vi "Alpha Ver 1.4.vi"() -> ()   [LabVIEW 2015]
uses:
  <instrlib>/Keithley 622x LV 2009/Configure/Source/Typedefs/KE622x -- Current Range.ctl
  <instrlib>/Keithley 622x LV 2009/Configure/Source/Typedefs/KE622x -- Current Ranges.ctl
  <instrlib>/Keithley 622x LV 2009/Typedefs/KE622x -- On Off Control.ctl
  <instrlib>/Keithley 622x LV 2009/Utility/Typedefs/KE622x -- Instrument Type.ctl
  <instrlib>/Keithley 622x LV 2009/Configure/Source/Typedefs/KE622x -- Voltage Limit.ctl
  <instrlib>/Keithley 2000/Public/Configure/Configure DC Volts.vi
  <userlib>/LV-Link3/PolySubVIs/DtCreateAinChan.vi
  <userlib>/LV-Link3/PolySubVIs/DtOLReadMultipleSingle.vi
  <instrlib>/Keithley 2000/Keithley 2000.lvlib
  <instrlib>/Keithley 622x LV 2009/Keithley 622x.lvlib
panel:
  out "XTC":i32
  out "SEN":i32
  in  "Time Delay":u16(ring) items=["0.1", "1", "3", "10", "30", "60"]
  out "FILE":refnum<file>
  out "Tick":u32
  in  "MULTIPLE GRAPHS Y":u16(ring) items=["Linear", "Log"]
  in  "MULTIPLE GRAPHS X":u16(ring) items=["Linear", "Log"]
  in  "TIME GRAPH Y":u16(ring) items=["Linear", "Log"]
  in  "TIME GRAPH X":u16(ring) items=["Linear", "Log"]
  in  "Lock-In, Y":dbl=1.0
  in  "Lock-In, X":dbl=1.0
  in  "DAQ A4":dbl=1.0
  in  "DAQ A3":dbl=1.0
  in  "DAQ A2":dbl=1.0
  in  "DAQ A1":dbl=1.0
  in  "DAQ A0":dbl=1.0
  in  "2000":dbl=1.0
  in  "Current":dbl=1000.0
  in  "Display Type 3":u16(ring)=3 items=["X %", "Y %", "X Calibrated", "Y Calibrated", "Mag %", "Mag Calibrated", "Phase Degrees", "Ratio", "ADC 1", "ADC 2", "ADC 3", "ADC 4 ", "Noise %", "Noise Calibrated", "Ref Frequency", "", ""]
  in  "Display Type 2":u16(ring)=2 items=["X %", "Y %", "X Calibrated", "Y Calibrated", "Mag %", "Mag Calibrated", "Phase Degrees", "Ratio", "ADC 1", "ADC 2", "ADC 3", "ADC 4 ", "Noise %", "Noise Calibrated", "Ref Frequency", "", ""]
  out "Units 3":string
  out "Display 3":dbl format="%.3f"
  out "Units 2":string
  out "Display 2":dbl format="%.3f"
  out "DAQ A4":dbl format="%#_13g"
  out "DAQ_clust":T1
  out "DAQ A3":dbl format="%#_13g"
  out "DAQ A2":dbl format="%#_13g"
  out "DAQ A1":dbl format="%#_13g"
  out "Real stop cur":dbl format="%#_13g"
  out "Real start cur":dbl format="%#_13g"
  in  "Stop cur prefix":u16(ring)=2
  in  "Start cur prefix":u16(ring)=2
  out "MULTIPLE GRAPHS":cluster{dbl[], dbl[]}[](graph)
  in  "X-Axis":T2(ring)
  in  "Range":u8(ring)=20 items=["100nV", "200nV", "500nV", "1µV", "2µV", "5µV", "10µV", "20µV", "50µV", "100µV", "200µV", "500µV", "1mV", "2mV", "5mV", "10mV", "20mV", "50mV", "100mV", "200mV", "500mV", "1V"]
  in  "Display Type copy":u16(ring)=3 items=["X %", "Y %", "X Calibrated", "Y Calibrated", "Mag %", "Mag Calibrated", "Phase Degrees", "Ratio", "ADC 1", "ADC 2", "ADC 3", "ADC 4 ", "Noise %", "Noise Calibrated", "Ref Frequency", "", ""]
  out "Units copy":string
  out "Display copy":dbl format="%.3f"
  out "Overload":bool
  out "Display":dbl format="%.3f"
  out "Units":string
  in  "Display Type":u16(ring)=2 items=["X %", "Y %", "X Calibrated", "Y Calibrated", "Mag %", "Mag Calibrated", "Phase Degrees", "Ratio", "ADC 1", "ADC 2", "ADC 3", "ADC 4 ", "Noise %", "Noise Calibrated", "Ref Frequency", "", ""]
  in  "Time Constant":u16(ring) items=["MIN", "1ms", "3ms", "10ms", "30ms", "100ms", "300ms", "1s", "3s", "10s", "30s", "100s", "300s"]
  in  "Slope":u8(ring) items=["6db/octave", "12dB/octave"]
  in  "Dynamic Reserve":u16(ring) items=["High Stability", "Normal", "High Reserve"]
  in  "Auto Sensitivity":bool
  in  "Auto Measure":bool
  out "6221_error_out":errorcluster
  out "2000_error_out":errorcluster
  out "5110_error_out":errorcluster
  out "Input Mode":i32(ring) items=[" Voltage Input (A or A-B) ", "Current Input 10E6 V/A", "Current Input 10E8 V/A"]
  out "5110":refnum<visa-resource-name>
  in  "GPIB Address":i8=11 min=1 max=32 step=1
  out "DAQ A0":dbl format="%#_13g"
  out "2000":dbl format="%#_13g"
  in  "Device":string(combo)
  in  "Number \nof points":i32=10
  in  "Folder\nprename":string
  out "TIME GRAPH":cluster{dbl[], dbl[]}[](graph)
  out "T0":u32
  out "LIMIT":bool
  out "LIMIT":bool
  out "Error Code":string
  in  "Comments":string
  out "2000":refnum<visa-resource-name>
  out "6221":refnum<visa-resource-name>
  out "Step  (A)":dbl=5e-05 format="%#_3p"
  in  "Stop\ncurrent (A)":dbl=2.0 format="%#_6p"
  in  "Start \ncurrent (A)":dbl=1.0 format="%#_6p"
  in  "Check For SCPI Errors? (T)":bool=TRUE
  out "Interlock Tripped?":bool
  out "Compliance?":bool
  in  "Turn Off Output \nIf Compliance?":bool=TRUE
  in  "Turning ON/OFF\ncurrent output":T3=enum."On"
  in  "Range Selection":T4={"Auto Range?"=TRUE, "Man / Selected\nRange"=enum."2nA"}
  # "FILE CONFIGURATION"
  # "ADMIN PANEL"
  # "MULTIPLIERS"
  # "SCALES"
  # "KEITHLEY 6221 CONFIGURATION (ADMIN ONLY)"
  # "KEITHLEY DAQ CONFIGURATION (ADMIN ONLY)"
  # "PRINCETON LOCK-IN AMP (ADMIN ONLY)"
  # "I don't know what the hell it is,\njust don't touch it"
  # "SENSITIVITY"
  # "INPUT CONFIGURATION"
  # "READINGS"
  # "START, STOP, STEP, CONFIGURATION"
  # "IF ON"
  # "Output Channels Time - Constant \nSlope & Dynamic Reserve"
  # "Compliance = Limiting output voltage\nThis switch determines if we want to switch \noff the current output if wee exceed compliance"
  # "SCALES"
  # "LOCK-IN READINGS"
  # "RIGHT DISPLAY"
  # "LEFT DISPLAY"
  # "There is a safe switch at \nthe back of the instrument \nThis indicator shows if it is on"
  # "You have hit a damn jackpot \nby exceeding the limited voltage\nCongrats"
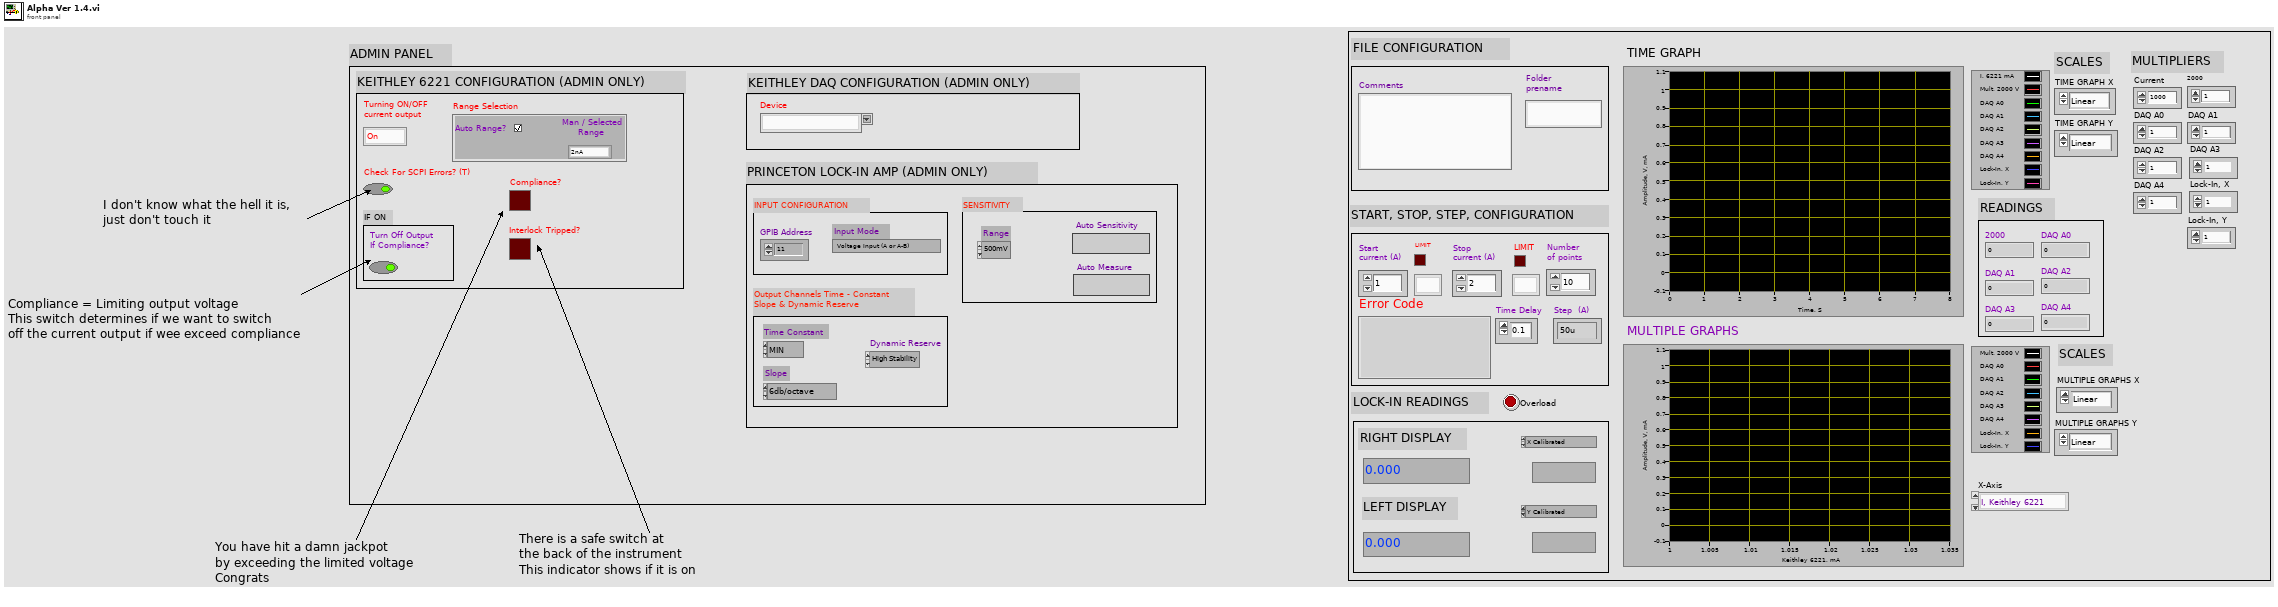
[diagram p1: front panel]
types:
  T1 = cluster{"Task out":i32, "Actual Number of Channels":u32, "error out":errorcluster}
  T2 = enum16{"I, Keithley 6221", "V, Keithley 2000", "V, Keithley DAQ A0", "V, Keithley DAQ A1", "V, Keithley DAQ A2", "V, Keithley DAQ A3", "V, Keithley DAQ A4", "V, Lock-In X", "V, Lock-In Y"}
  T3 = typedef "Keithley 622x.lvlib/KE622x -- On Off Control.ctl" = enum16{"Off", "On"}
  T4 = typedef "Keithley 622x.lvlib/KE622x -- Current Range.ctl" = cluster{"Auto Range?":bool, "Man / Selected\nRange":T5}
  T5 = typedef "Keithley 622x.lvlib/KE622x -- Current Ranges.ctl" = enum16{"2nA", "20nA", "200nA", "2uA", "20uA", "200uA", "2mA", "20mA", "100mA"}
  T6 = typedef "Keithley 622x.lvlib/KE622x -- Instrument Type.ctl" = enum16{"KE6220", "KE6221"}
  T7 = typedef "Keithley 622x.lvlib/KE622x -- Voltage Limit.ctl" = dbl
  T8 = cluster{"Task out":i32, "error out":errorcluster}
  T9 = cluster{dbl, dbl, dbl, dbl, dbl, "Measurement":dbl}
  T10 = cluster{dbl[], dbl[], dbl[], dbl[], dbl[], dbl[], dbl[], dbl[], dbl[], dbl[]}
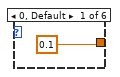
[diagram p2: hidden frame]
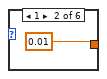
[diagram p3: hidden frame]
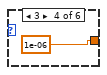
[diagram p4: hidden frame]
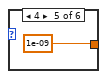
[diagram p5: hidden frame]
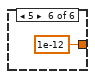
[diagram p6: hidden frame]
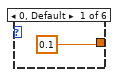
[diagram p7: hidden frame]
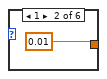
[diagram p8: hidden frame]
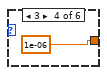
[diagram p9: hidden frame]
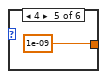
[diagram p10: hidden frame]
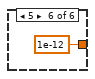
[diagram p11: hidden frame]
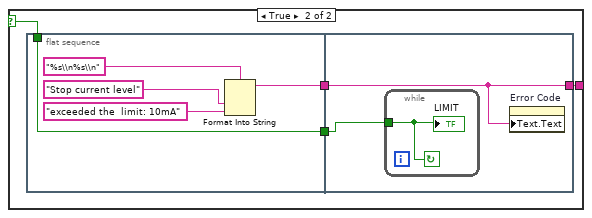
[diagram p12: hidden frame]
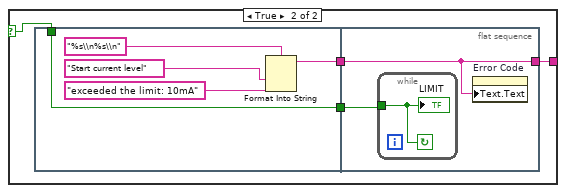
[diagram p13: hidden frame]
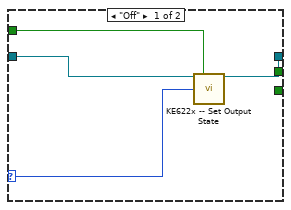
[diagram p14: hidden frame]
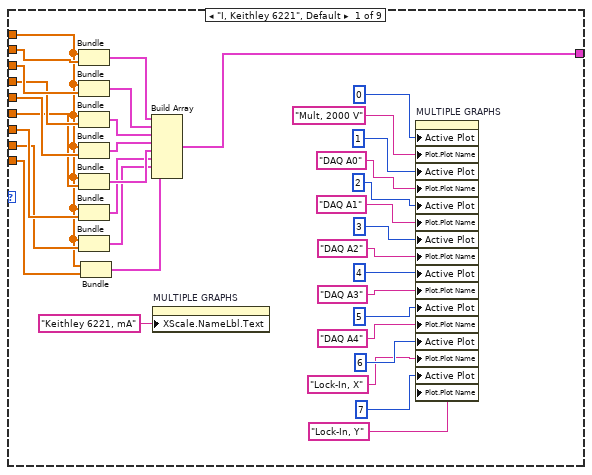
[diagram p15: hidden frame]
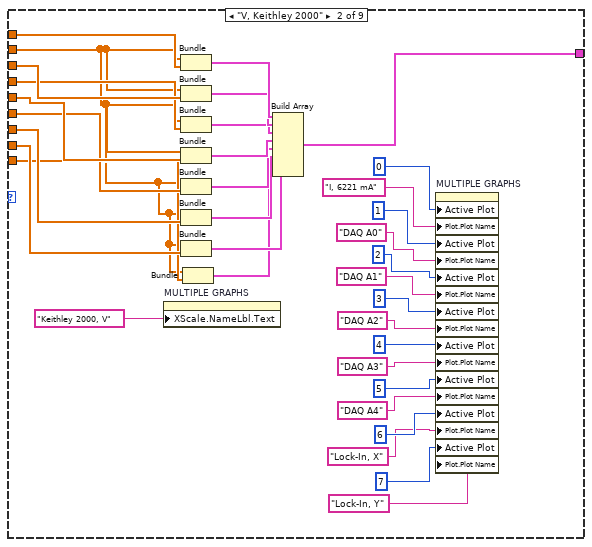
[diagram p16: hidden frame]
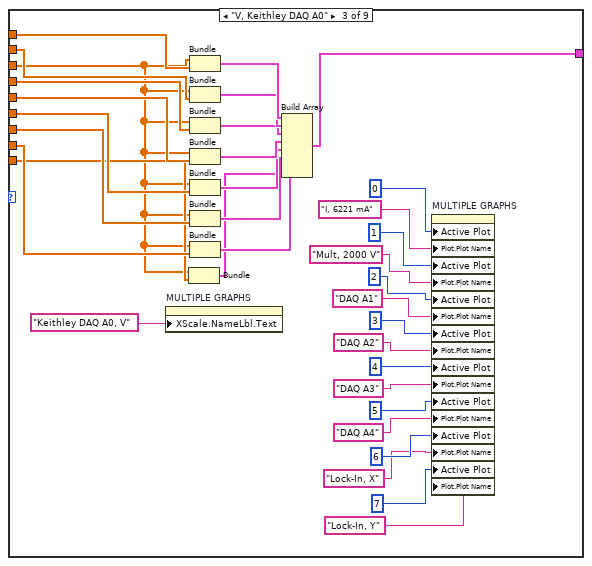
[diagram p17: hidden frame]
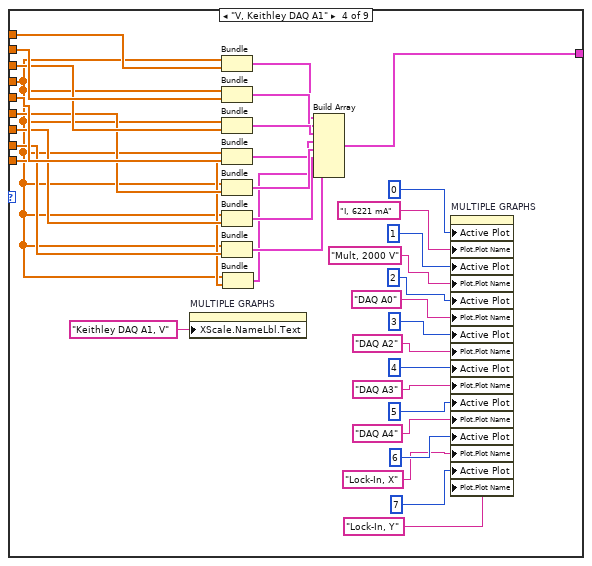
[diagram p18: hidden frame]
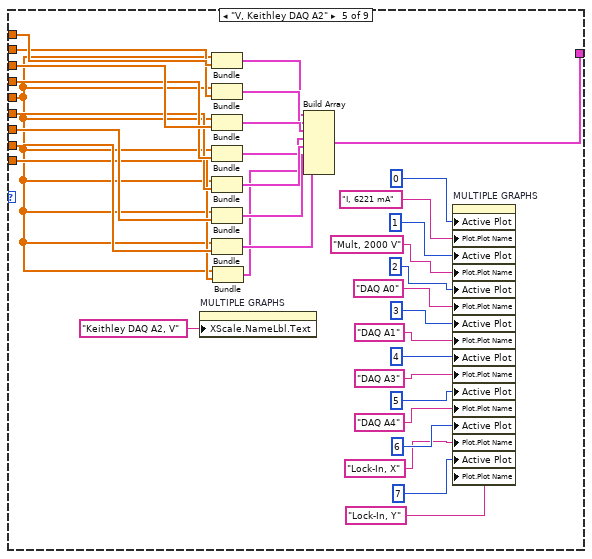
[diagram p19: hidden frame]
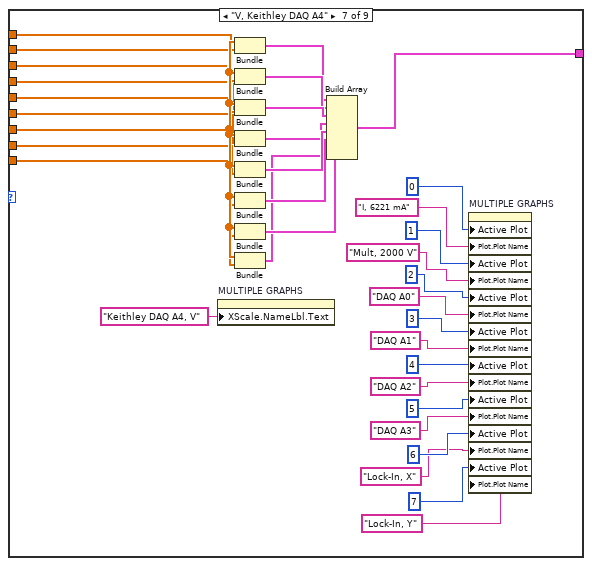
[diagram p20: hidden frame]
diagram:
  n1 = flat-sequence {
    tunnel: [w177] -> w7
    tunnel: [w176] -> w6
    tunnel: [w175] -> w5
    tunnel: [w174] -> w4
    tunnel: [w173] -> w3
    tunnel: [w172] -> w2
    tunnel: [w161] -> w1
    tunnel: w7 -> [w1027]
    tunnel: w6 -> [w1026]
    tunnel: w5 -> [w1025]
    tunnel: w4 -> [w1024]
    tunnel: w3 -> [w1023]
    tunnel: w2 -> [w1022]
    tunnel: w1 -> [w1021]
    frame #0 {
      # "File configuration"
      # "Start, Stop, Step"
      # "Initializing instruments"
      n2 = flat-sequence {
        frame #0 {
          w15 = TRUE  # reset
          w14 = FALSE  # ID query
          # "Initialize Lock-In 5110"
          # "Initialize Keithley 2000"
          # "Initialize Keithley 6221"
          n3 = call <instrlib>:"Initialize.vi"("VISA resource name"=refnum<visa-resource-name> "KEITHLEY_MULTIMETER") -> ("VISA resource name out"=w19:refnum<visa-resource-name>)  [unwired: 17 in, 1 out]
          n4 = call <instrlib>:"Initialize.vi"("VISA resource name"=refnum<visa-resource-name> "KEITHLEY_DC_AC_CURRENT_SOURCE", "Error Queue Option"=enum16{"Clear Error Queue", "Error Query"}."Clear Error Queue", "Instrument Type"=KE622x_--_Instrument_Type."KE6221") -> ("VISA resource name out"=→"6221":refnum<visa-resource-name>, "error out"=→"6221_error_out":errorcluster)  [unwired: 11 in]
          n5 = call "SR51XX Initialize"("VISA session (for class)"=refnum<visa-resource-name> "LOCK_IN_5110_PRINCETON", "Interface"=FALSE, "ID query"=w14, "GPIB Address"="GPIB Address", "reset"=w15) -> ("VISA session"=→"5110":refnum<visa-resource-name>, "error out"=→"5110_error_out":errorcluster)  [unwired: 8 in, 1 out]
          n6 = call-poly <instrlib>:"Configure Measurement.vi"("VISA resource name"=w19) -> ("VISA resource name out"=→"2000":refnum<visa-resource-name>, "error out"=→"2000_error_out":errorcluster)  [unwired: 17 in]
        }
        frame #1 {
          # "Initialize Keithley DAQ \n(getting board name)"
          n7 = call <userlib>:"DtOLGetBoardNames.vi"() -> ("Number of boards"=w24:u32)  [unwired: 9 in, 2 out]
          n8 = Initialize Array("", w24) -> (w26:string[])
          n9 = for {
            N: w24 -> [_]
            shift-right: [w32] -> w29
            shift-left: w26 -> [w33]
            i -> [w31]
            n10 = Add(x=1, y=w31) -> (x+y=w35:i32)
            n11 = call <userlib>:"DtOLGetBoardNames.vi"("Select Board"=w35) -> ("Board Name"=w30:string)  [unwired: 8 in, 2 out]
            n12 = Replace Array Subset(array=w33, new element=w30, index=w31) -> (w32:string[])
          }
          n13 = Index Array(array=w29, index=0) -> (element=w28:string)
          n14 = property on="Device" class="CmbBox"("Strings[]"=w29, "Value"=w28) -> ()  [unwired: 2 in, 2 out]
        }
        frame #2 {
          # "Calculating steps by number\nof points"
          # "Putting in a loop \ninstead of \"STOP\""
          n15 = local read "Real stop cur"() -> (w52:dbl)
          n16 = local read "Real start cur"() -> (w53:dbl)
          n17 = case shown="2" "Start cur prefix" {
            tunnel: [0.1 0.01 0.001 1e-06 1e-09 1e-12] -> w41
            frame 0, Default {
            }
            frame 1 {
            }
            frame 2 {
            }
            frame 3 {
            }
            frame 4 {
            }
            frame 5 {
            }
          }
          n18 = case shown="2" "Stop cur prefix" {
            tunnel: [0.1 0.01 0.001 1e-06 1e-09 1e-12] -> w39
            frame 0, Default {
            }
            frame 1 {
            }
            frame 2 {
            }
            frame 3 {
            }
            frame 4 {
            }
            frame 5 {
            }
          }
          n19 = Subtract(x=w52, y=w53) -> (x-y=w55:dbl)
          n20 = Multiply(x=w41, y="Start \ncurrent (A)") -> (x*y=w37:dbl)
          "Real start cur" <- w37
          n21 = Divide(x=w55, y="Number \nof points") -> (x/y=→"Step  (A)":dbl)
          n22 = Multiply(x=w39, y="Stop\ncurrent (A)") -> (x*y=w36:dbl)
          "Real stop cur" <- w36
          n23 = Greater?(x=w36, y=T7 0.01) -> (0:w47:bool)
          n24 = Greater?(x=w37, y=T7 0.01) -> (0:w46:bool)
          n25 = case shown="False" w47 {
            selector: w47 -> [_ w71]
            tunnel: [w68 w74] -> w49
            frame False {
              n26 = Format Into String(format string="%s\\n", "Start current level is OK" ("false string")) -> (resulting string=w68:string)  [unwired: 2 in, 1 out]
            }
            frame True {
              n27 = flat-sequence {
                tunnel: [w76] -> w73
                tunnel: [w75] -> w72
                tunnel: w71 -> [w75]
                tunnel: [w80] -> w74
                tunnel: w73 -> [w80]
                tunnel: w72 -> [w81]
                frame #0 {
                  n28 = Format Into String(format string="%s\\n%s\\n", "Stop current level" ("String"), "exceeded the  limit: 10mA" ("input 2")) -> (resulting string=w76:string)  [unwired: 2 in, 1 out]
                }
                frame #1 {
                  n29 = while {
                    tunnel: w81 -> [w82]
                    stop <- w82 continue-if-true
                    "LIMIT" <- w82
                  }
                  n30 = property on="Error Code" class="Str"("Text.Text"=w80) -> ()  [unwired: 2 in, 2 out]
                }
              }
            }
          }
          n31 = case shown="False" w46 {
            selector: w46 -> [_ w87]
            tunnel: [w83 w89] -> w48
            frame False {
              n32 = Format Into String(format string="%s\\n", "Start current level is OK" ("false string")) -> (resulting string=w83:string)  [unwired: 2 in, 1 out]
            }
            frame True {
              n33 = flat-sequence {
                tunnel: [w91] -> w88
                tunnel: w87 -> [w90]
                tunnel: [w90] -> w86
                tunnel: [w95] -> w89
                tunnel: w88 -> [w95]
                tunnel: w86 -> [w96]
                frame #0 {
                  n34 = Format Into String(format string="%s\\n%s\\n", "Start current level" ("String"), "exceeded the limit: 10mA" ("input 2")) -> (resulting string=w91:string)  [unwired: 2 in, 1 out]
                }
                frame #1 {
                  n35 = while {
                    tunnel: w96 -> [w97]
                    stop <- w97 continue-if-true
                    "LIMIT" <- w97
                  }
                  n36 = property on="Error Code" class="Str"("Text.Text"=w95) -> ()  [unwired: 2 in, 2 out]
                }
              }
            }
          }
          n37 = Concatenate Strings(w48, w49) -> (→"Error Code":string)
        }
        frame #3 {
          # "Adding headlines"
          # "Creating folder&file"
          # "Creating comments"
          # "Writing instr params"
          n38 = local read "5110"() -> (w103:refnum<visa-resource-name>)
          n39 = local read "Real stop cur"() -> (w101:dbl)
          n40 = local read "Real start cur"() -> (w102:dbl)
          n41 = call "folder_creation.vi"("Name"="Folder\nprename") -> ("String"=w119:string)
          n42 = call "file_creation.vi"("String"=w119) -> ("refnum out"=w104:refnum<file>)
          "FILE" <- w104
          n43 = call "com_inst.vi"("Stop current"=w101, "Start current"=w102, "VISA session (for class)"=w103) -> ("XTC"=→"XTC":i32, "SEN"=→"SEN":i32, "concatenated string"=w100:string)
          n44 = Format Into String(format string="# %s\\n", initial string=w104, "Comments") -> (resulting string=w106:refnum<file>)  [unwired: 1 in, 1 out]
          n45 = Format Into String(format string="# %s\\n", initial string=w106, w100) -> (resulting string=w105:refnum<file>)  [unwired: 1 in, 1 out]
          n46 = Format Into String(format string="# %-6s  %-12s %-12s %-14s %-12s %-14s %-12s %-12s %-14s%-14s\\n", initial string=w105, "t, ms" ("input 3"), "2000, V" ("input 1"), "DAQ A0, V" ("input 2"), "DAQ A1, V" ("input 2"), "DAQ A2, V" ("input 2"), "DAQ A3, V" ("input 2"), "DAQ A4, V" ("input 2"), "5110_X, V" ("input 3"), "5110_Y, V " ("input 3"), "6221, A" ("input 3")) -> ()  [unwired: 1 in, 2 out]
        }
        frame #4 {
          # "Time Intit"
          n47 = Wait Until Next ms Multiple(millisecond multiple=u32 1000) -> (millisecond timer value=→"T0":u32)
        }
      }
    }
    frame #1 {
      # "Configuring Keithley DAQ just before measuments"
      # "Configuring Keithley 6221 just before measuments"
      n48 = flat-sequence {
        tunnel: [w135] -> w125
        tunnel: [w153] -> _
        tunnel: [w155] -> _
        tunnel: w125 -> [w154]
        frame #0 {
          # "Current range \nselection check"
          # "Checking for compliance\nand interlock errors"
          n49 = local read "6221"() -> (w138:refnum<visa-resource-name>)
          n50 = call <instrlib>:"KE622x -- Set Current Range.vi"("Resource In"=w138, "Current Range In"="Range Selection", "Read Back Set Values? (T)"=FALSE) -> ("Resource Out (dupl)"=w143:refnum<visa-resource-name>)  [unwired: 10 in, 2 out]
          n51 = case shown="\"On\"" "Turning ON/OFF\ncurrent output" {
            selector: "Turning ON/OFF\ncurrent output" -> [w147 _]
            tunnel: [_ w151] -> w141
            tunnel: [_ w150] -> w142
            tunnel: "Check For SCPI Errors? (T)" -> [w146 _]
            tunnel: w143 -> [w144 w149]
            tunnel: [w145 w148] -> w135
            frame "Off" {
              n52 = call <instrlib>:"KE622x -- Set Output State.vi"("Resource In"=w144, "Check For SCPI Errors? (T)"=w146, "Output State"=w147) -> ("Resource Out (dupl)"=w145:refnum<visa-resource-name>)  [unwired: 11 in, 1 out]
            }
            frame "On" {
              n53 = call <instrlib>:"KE622x -- Turn Output On And Check For Errors.vi"("Resource In"=w149, "Turn Off Output If Compliance?"="Turn Off Output \nIf Compliance?") -> ("Resource Out (dupl)"=w148:refnum<visa-resource-name>, "Interlock Tripped?"=w151:bool, "Compliance?"=w150:bool)  [unwired: 10 in, 1 out]
            }
          }
          "Interlock Tripped?" <- w141
          "Compliance?" <- w142
        }
        frame #1 {
          # "Setting start current"
          n54 = local read "Real start cur"() -> (w153:dbl)
          n55 = Wait (ms)(milliseconds to wait=u32 100) -> ()  [unwired: 1 out]
          n56 = call <instrlib>:"KE622x -- Set Current Level.vi"("Resource In"=w154, "Current Level (A) In"=w153) -> ("Resource Out (dupl)"=w155:refnum<visa-resource-name>)  [unwired: 12 in, 1 out]
        }
      }
      n57 = flat-sequence {
        frame #0 {
          w130 = 100 items=["SingleEnded"=100, "Differential"=101] ("Channel Type")
          # "Configure the input channel"
          n58 = call-poly <userlib>:"DtOLCreateTask.vi"("Channel Type"=w130, "Range Min"=-10.0, "Range Max"=10.0, "Board Name"="Device", "Channel"="0:4" ("Channels")) -> ("Task out"=w129:i32, "Actual Number of Channels"=w128:u32, "error out"=w127:errorcluster)  [unwired: 8 in]
          n59 = Bundle("Task out"=w129, "Actual Number of Channels"=w128, "error out"=w127) -> (→"DAQ_clust":T1)  [unwired: 1 in]
        }
      }
    }
    frame #2 {
      n60 = local read "5110"() -> (w168:refnum<visa-resource-name>)
      n61 = local read "2000"() -> (w167:refnum<visa-resource-name>)
      n62 = local read "6221"() -> (w166:refnum<visa-resource-name>)
      n63 = local read "5110_error_out"() -> (w165:errorcluster)
      n64 = local read "6221_error_out"() -> (w164:errorcluster)
      n65 = local read "2000_error_out"() -> (w163:errorcluster)
      n66 = local read "DAQ_clust"() -> (w162:T1)
      n67 = while {
        shift-right: [w330] -> _
        shift-left: dbl[] [] -> [w455]
        shift-right: [w331] -> _
        shift-left: i32[] [] -> [w454]
        tunnel: w167 -> [w452]
        tunnel: w166 -> [w451]
        shift-right: [w288] -> _
        shift-left: dbl[] [] -> [w445]
        tunnel: [w444] -> w177
        tunnel: [w443] -> w176
        tunnel: [w441] -> w175
        tunnel: [w439] -> w174
        tunnel: w168 -> [w437]
        tunnel: w165 -> [w436]
        tunnel: w164 -> [w428]
        tunnel: w163 -> [w427]
        tunnel: [w392] -> w173
        tunnel: [w390] -> w172
        shift-right: [w290] -> _
        shift-left: dbl[] [] -> [w389]
        shift-right: [w291] -> _
        shift-left: dbl[] [] -> [w388]
        shift-right: [w332] -> _
        shift-left: dbl[] [] -> [w385]
        tunnel: w162 -> [w345]
        tunnel: [w344] -> w161
        shift-right: [w329] -> _
        shift-left: dbl[] [] -> [w343]
        shift-right: [w328] -> _
        shift-left: dbl[] [] -> [w342]
        shift-right: [w327] -> _
        shift-left: dbl[] [] -> [w341]
        shift-right: [w289] -> _
        shift-left: dbl[] [] -> [w293]
        i -> [w429]
        stop <- w446 stop-if-true
        # "V, DAQ A4"
        # "V, DAQ A3"
        # "V, DAQ A2"
        # "V, DAQ A1"
        # "Y-V, 5110"
        # "X-V, 5110"
        # "I, 6221"
        # "Config delay"
        # "Control subVI 5110"
        # "Read config 5110"
        # "Measurement config 5110"
        # "Time config 5110"
        # "Configuring Right Display 5110"
        # "Configuring Left Display 5110"
        # "Setting 6221 current"
        # "Delay before measuremens"
        # "Getting the data from DAQ and 2000"
        # "Changing input current"
        # "Time"
        # "V, DAQ A0"
        # "V, 2000"
        n68 = local read "T0"() -> (w453:u32)
        n69 = Quotient & Remainder(x=w429, y=10) -> (floor(x/y)=w434:i32)  [unwired: 1 out]
        n70 = Equal?(x=0, y=w429) -> (x = y?=w431:bool)
        n71 = Subtract(x=w420, y=w453) -> (x-y=w354:u32)
        n72 = Equal?(x=1, y=w434) -> (x = y?=w430:bool)
        n73 = Divide(x=w354, y=u32 1000) -> (x/y=w355:dbl)
        n74 = local read "FILE"() -> (w193:refnum<file>)
        n75 = flat-sequence {
          tunnel: w452 -> [w780]
          tunnel: [w780] -> w384
          tunnel: w451 -> [w779]
          tunnel: [w779] -> w382
          tunnel: w437 -> [w778]
          tunnel: [w778] -> w380
          tunnel: [w777] -> w378
          tunnel: w436 -> [w777]
          tunnel: w431 -> [w776]
          tunnel: [w776] -> w376
          tunnel: w430 -> [w775]
          tunnel: [w775] -> w374
          tunnel: w428 -> [w774]
          tunnel: [w774] -> w372
          tunnel: w427 -> [w773]
          tunnel: [w773] -> w370
          tunnel: [w771] -> w420
          tunnel: [w772] -> w346
          tunnel: w345 -> [w772]
          tunnel: w384 -> [w795]
          tunnel: [w795] -> w383
          tunnel: w382 -> [w794]
          tunnel: [w794] -> w381
          tunnel: w380 -> [w793]
          tunnel: [w793] -> w379
          tunnel: w378 -> [w792]
          tunnel: [w792] -> w377
          tunnel: w376 -> [w791]
          tunnel: [w791] -> w375
          tunnel: w374 -> [w790]
          tunnel: [w790] -> w373
          tunnel: w372 -> [w789]
          tunnel: [w789] -> w371
          tunnel: w370 -> [w788]
          tunnel: [w788] -> w369
          tunnel: [w781] -> w347
          tunnel: w346 -> [w781]
          tunnel: w383 -> [w808]
          tunnel: [w808] -> w419
          tunnel: w381 -> [w807]
          tunnel: [w807] -> w418
          tunnel: w379 -> [w806]
          tunnel: w377 -> [w803]
          tunnel: [w802] -> w417
          tunnel: [w801] -> w416
          tunnel: w375 -> [w800]
          tunnel: [w800] -> w415
          tunnel: w373 -> [w799]
          tunnel: w371 -> [w798]
          tunnel: [w798] -> w414
          tunnel: w369 -> [w797]
          tunnel: [w797] -> w413
          tunnel: [w796] -> w348
          tunnel: w347 -> [w796]
          tunnel: w419 -> [w833]
          tunnel: [w833] -> w412
          tunnel: w418 -> [w832]
          tunnel: [w832] -> w411
          tunnel: w417 -> [w829]
          tunnel: [w828] -> w410
          tunnel: w416 -> [w827]
          tunnel: [w826] -> w409
          tunnel: w415 -> [w824]
          tunnel: [w824] -> w408
          tunnel: w414 -> [w831]
          tunnel: [w831] -> w407
          tunnel: w413 -> [w830]
          tunnel: [w830] -> w406
          tunnel: ["Auto Measure"] -> w405
          tunnel: ["Auto Sensitivity"] -> w404
          tunnel: [w819] -> w403
          tunnel: [w816] -> w349
          tunnel: w348 -> [w816]
          tunnel: w412 -> [w852]
          tunnel: [w852] -> w368
          tunnel: w411 -> [w851]
          tunnel: [w851] -> w367
          tunnel: w410 -> [w844]
          tunnel: w409 -> [w842]
          tunnel: [w841] -> w366
          tunnel: w408 -> [w848]
          tunnel: [w848] -> w365
          tunnel: w407 -> [w850]
          tunnel: [w850] -> w364
          tunnel: w406 -> [w849]
          tunnel: [w849] -> w363
          tunnel: w405 -> [w846]
          tunnel: [w846] -> w362
          tunnel: w404 -> [w847]
          tunnel: [w847] -> w361
          tunnel: w403 -> [w837]
          tunnel: [w837] -> w360
          tunnel: [w843] -> w359
          tunnel: ["Time Constant"] -> w358
          tunnel: ["Slope"] -> w357
          tunnel: [w834] -> w350
          tunnel: w349 -> [w834]
          tunnel: [w874] -> w286
          tunnel: [w873] -> w285
          tunnel: [w859] -> w284
          tunnel: [w872] -> w283
          tunnel: [w871] -> w282
          tunnel: [w870] -> w281
          tunnel: [w869] -> w280
          tunnel: [w868] -> w279
          tunnel: [w861] -> w278
          tunnel: [w864] -> w277
          tunnel: [w862] -> w276
          tunnel: [w867] -> w275
          tunnel: w357 -> [w867]
          tunnel: w358 -> [w862]
          tunnel: w359 -> [w865]
          tunnel: w360 -> [w861]
          tunnel: w361 -> [w868]
          tunnel: w362 -> [w869]
          tunnel: w363 -> [w870]
          tunnel: w364 -> [w871]
          tunnel: w365 -> [w872]
          tunnel: w366 -> [w860]
          tunnel: w367 -> [w873]
          tunnel: w368 -> [w874]
          tunnel: [w853] -> w274
          tunnel: w350 -> [w853]
          tunnel: w286 -> [w897]
          tunnel: [w897] -> w273
          tunnel: w285 -> [w896]
          tunnel: [w896] -> w271
          tunnel: w284 -> [w888]
          tunnel: [w887] -> w269
          tunnel: w283 -> [w895]
          tunnel: [w895] -> w267
          tunnel: w282 -> [w894]
          tunnel: [w894] -> w265
          tunnel: w281 -> [w893]
          tunnel: [w893] -> w263
          tunnel: w280 -> [w892]
          tunnel: [w892] -> w261
          tunnel: w279 -> [w891]
          tunnel: [w891] -> w259
          tunnel: w278 -> [w882]
          tunnel: [w882] -> w257
          tunnel: w277 -> [w889]
          tunnel: [w886] -> w255
          tunnel: w276 -> [w884]
          tunnel: [w884] -> w253
          tunnel: w275 -> [w881]
          tunnel: [w881] -> w251
          tunnel: w274 -> [w890]
          tunnel: [w890] -> w249
          tunnel: [w877] -> w246
          tunnel: w273 -> [w920]
          tunnel: [w920] -> w272
          tunnel: w271 -> [w919]
          tunnel: [w919] -> w270
          tunnel: w269 -> [w910]
          tunnel: [w909] -> w268
          tunnel: w267 -> [w918]
          tunnel: [w918] -> w266
          tunnel: w265 -> [w917]
          tunnel: [w917] -> w264
          tunnel: w263 -> [w916]
          tunnel: [w916] -> w262
          tunnel: w261 -> [w915]
          tunnel: [w915] -> w260
          tunnel: w259 -> [w914]
          tunnel: [w914] -> w258
          tunnel: w257 -> [w905]
          tunnel: [w905] -> w256
          tunnel: w255 -> [w912]
          tunnel: [w911] -> w254
          tunnel: w253 -> [w907]
          tunnel: [w907] -> w252
          tunnel: w251 -> [w904]
          tunnel: [w904] -> w250
          tunnel: w249 -> [w913]
          tunnel: [w913] -> w248
          tunnel: [w900] -> w247
          tunnel: w272 -> [w942]
          tunnel: [w942] -> w402
          tunnel: w270 -> [w941]
          tunnel: [w941] -> w401
          tunnel: w268 -> [w928]
          tunnel: w266 -> [w940]
          tunnel: [w940] -> w400
          tunnel: w264 -> [w939]
          tunnel: [w939] -> w399
          tunnel: w262 -> [w938]
          tunnel: [w938] -> w398
          tunnel: w260 -> [w937]
          tunnel: [w937] -> w397
          tunnel: w258 -> [w936]
          tunnel: [w936] -> w396
          tunnel: w256 -> [w929]
          tunnel: w254 -> [w926]
          tunnel: [w925] -> w395
          tunnel: w252 -> [w930]
          tunnel: w250 -> [w931]
          tunnel: [w927] -> w394
          tunnel: [w924] -> w393
          tunnel: [w921] -> w351
          tunnel: w248 -> [w921]
          tunnel: [w946] -> w450
          tunnel: w429 -> [w954]
          tunnel: [w950] -> w446
          tunnel: [w944] -> w448
          tunnel: [w952] -> w447
          tunnel: [w949] -> w426
          tunnel: [w948] -> w425
          tunnel: [w947] -> w424
          tunnel: [w945] -> w423
          tunnel: [w944] -> w340
          tunnel: w393 -> [_]
          tunnel: w394 -> [w947]
          tunnel: w395 -> [w945]
          tunnel: w396 -> [_]
          tunnel: w397 -> [_]
          tunnel: w398 -> [w949]
          tunnel: w399 -> [w948]
          tunnel: w400 -> [_]
          tunnel: w401 -> [w952]
          tunnel: w402 -> [w946]
          tunnel: [w943] -> w352
          tunnel: w351 -> [w943]
          tunnel: w450 -> [w967]
          tunnel: [w967] -> w449
          tunnel: w448 -> [w966]
          tunnel: w447 -> [w965]
          tunnel: [w964] -> w442
          tunnel: [w963] -> w440
          tunnel: w426 -> [w961]
          tunnel: w425 -> [w962]
          tunnel: w424 -> [w959]
          tunnel: w423 -> [w960]
          tunnel: [w961] -> w422
          tunnel: [w960] -> w421
          tunnel: [w959] -> w391
          tunnel: [w958] -> w353
          tunnel: w352 -> [w958]
          tunnel: [w1004] -> w315
          tunnel: [w971] -> w314
          tunnel: [w1003] -> w313
          tunnel: [w1002] -> w312
          tunnel: [w1001] -> w311
          tunnel: [w1000] -> w310
          tunnel: [w972] -> w309
          tunnel: [w1004] -> w308
          tunnel: [w999] -> w307
          tunnel: [w998] -> w306
          tunnel: [w997] -> w305
          tunnel: [w970] -> w304
          tunnel: [w969] -> w303
          tunnel: [w968] -> w302
          tunnel: w353 -> [w994]
          tunnel: w391 -> [w998]
          tunnel: w421 -> [w999]
          tunnel: w422 -> [w995]
          tunnel: w440 -> [w1000]
          tunnel: w442 -> [w1001]
          tunnel: w449 -> [w996]
          tunnel: [w1008] -> w344
          tunnel: [w1009] -> w390
          tunnel: [w1010] -> w392
          tunnel: [w1011] -> w438
          tunnel: [w1012] -> w301
          tunnel: [w1013] -> w439
          tunnel: [w1014] -> w441
          tunnel: [w1015] -> w443
          tunnel: [w1016] -> w444
          tunnel: [w1017] -> w300
          tunnel: [w1018] -> w296
          tunnel: w315 -> [w1018]
          tunnel: w314 -> [w1017]
          tunnel: w313 -> [w1016]
          tunnel: w312 -> [w1015]
          tunnel: w311 -> [w1014]
          tunnel: w310 -> [w1013]
          tunnel: w309 -> [w1012]
          tunnel: w308 -> [w1011]
          tunnel: w307 -> [w1010]
          tunnel: w306 -> [w1009]
          tunnel: w305 -> [w1008]
          tunnel: [w1007] -> w299
          tunnel: w304 -> [w1007]
          tunnel: [w1006] -> w298
          tunnel: w303 -> [w1006]
          tunnel: w302 -> [w1005]
          tunnel: [w1005] -> w297
          frame #0 {
            n76 = Tick Count (ms)() -> (millisecond timer value=w771:u32)
            "Tick" <- w771
          }
          frame #1 {
            n77 = control-ref of="Range"() -> (w787:refnum<vi>)
            n78 = control-ref of="Auto Sensitivity"() -> (w786:refnum<vi>)
            n79 = control-ref of="Auto Measure"() -> (w785:refnum<vi>)
            n80 = control-ref of="Time Constant"() -> (w782:refnum<vi>)
            n81 = control-ref of="Slope"() -> (w783:refnum<vi>)
            n82 = control-ref of="Dynamic Reserve"() -> (w784:refnum<vi>)
            n83 = call "cont_ver_1.0.vi"("Dynamic Reserve"=w784, "Slope"=w783, "Time Constant"=w782, "Auto Measure"=w785, "Auto Sensitivity"=w786, "Range"=w787) -> ()
          }
          frame #2 {
            n84 = case shown="False" w799 {
              tunnel: w806 -> [w810 w815]
              tunnel: [w809 w813] -> w805
              tunnel: [w810 w812] -> w804
              tunnel: w803 -> [w809 w811]
              frame False {
              }
              frame True {
                n85 = call "SR51XX Read Preamp Input Mode"("VISA session (for class)"=w815, "error in (no error)"=w811) -> ("VISA session"=w812:refnum<visa-resource-name>, "Input Mode"=w814:i32, "error out"=w813:errorcluster)  [unwired: 15 in]
                n86 = local write "Input Mode"(w814) -> ()
              }
            }
            n87 = call "SR51XX Configure Signal Channel Input"("VISA session (for class)"=w804, "error in (no error)"=w805, "Update"=w800) -> ("VISA session"=w802:refnum<visa-resource-name>, "error out"=w801:errorcluster)  [unwired: 15 in]
          }
          frame #3 {
            n88 = local read "Input Mode"() -> (w825:i32)
            n89 = call "SR51XX Configure Sensitivity"("VISA session (for class)"=w829, "Input Mode"=w825, "Range"="Range", "error in (no error)"=w827, "Auto Sensitivity"="Auto Sensitivity", "Auto Measure"="Auto Measure", "Update"=w824) -> ("Range Annotations Out[]"=w817:string[], "VISA session"=w828:refnum<visa-resource-name>, "Auto Sensitivity out"=w821:bool, "Auto Measure out"=w820:bool, "Range Out"=w819:u8, "error out"=w826:errorcluster)  [unwired: 7 in]
            n90 = property on="Range" class="Ring (strict)"("Strings []"=w817) -> ()  [unwired: 2 in, 2 out]
            n91 = local write "Auto Sensitivity"(w821) -> ()
            n92 = local write "Auto Measure"(w820) -> ()
            n93 = local write "Range"(w819) -> ()
          }
          frame #4 {
            n94 = Or(x=w847, y=w846) -> (x .or. y?=w845:bool)
            n95 = call "SR51XX Configure Output Channels - Slope, TC and Dyn Reserve"("VISA session (for class)"=w844, "Time Constant"="Time Constant", "Slope"="Slope", "Check TC"=w845, "Dynamic Reserve"="Dynamic Reserve", "error in (no error)"=w842, "Range"=w837, "Update"=w848) -> ("VISA session"=w843:refnum<visa-resource-name>, "Slope Out"=w838:u8, "Time Constant Out"=w839:u16, "error out"=w841:errorcluster)  [unwired: 8 in]
            n96 = local write "Slope"(w838) -> ()
            n97 = local write "Time Constant"(w839) -> ()
          }
          frame #5 {
            n98 = local read "Input Mode"() -> (w866:i32)
            n99 = call "SR5110 Read Output"("VISA session (for class)"=w865, "Input Mode"=w866, "Time Constant"=w862, "Display Type"="Display Type", "Range"=w861, "error in (no error)"=w860, "Slope"=w867) -> ("Units"=→"Units":string, "Display Precision"=w858:i32, "Display"=→"Display":dbl, "VISA session"=w864:refnum<visa-resource-name>, "Available Display Types Out"=w857:string[], "Overload"=→"Overload":bool, "error out"=w859:errorcluster)  [unwired: 4 in, 2 out]
            n100 = property on="Display Type" class="Ring (strict)"("Strings []"=w857) -> ()  [unwired: 2 in, 2 out]
            n101 = property on="Display" class="DigNum (strict)"("Precision"=w858) -> ()  [unwired: 2 in, 2 out]
          }
          frame #6 {
            n102 = local read "Input Mode"() -> (w885:i32)
            n103 = call "SR5110 Read Output"("VISA session (for class)"=w889, "Input Mode"=w885, "Time Constant"=w884, "Display Type"="Display Type 2", "Range"=w882, "error in (no error)"=w888, "Slope"=w881) -> ("Units"=w875:string, "Display Precision"=w879:i32, "Display"=w876:dbl, "VISA session"=w886:refnum<visa-resource-name>, "Available Display Types Out"=w880:string[], "error out"=w887:errorcluster)  [unwired: 4 in, 3 out]
            "Display 2" <- w876
            "Units 2" <- w875
            n104 = call "pref_to_num.vi"("string"=w875) -> ("Numeric"=w878:dbl)
            n105 = property on="Display Type 2" class="Ring (strict)"("Strings []"=w880) -> ()  [unwired: 2 in, 2 out]
            n106 = property on="Display 2" class="DigNum (strict)"("Precision"=w879) -> ()  [unwired: 2 in, 2 out]
            n107 = Multiply(x=w878, y=w876) -> (x*y=w877:dbl)
          }
          frame #7 {
            n108 = local read "Input Mode"() -> (w908:i32)
            n109 = call "SR5110 Read Output"("VISA session (for class)"=w912, "Input Mode"=w908, "Time Constant"=w907, "Display Type"="Display Type 3", "Range"=w905, "error in (no error)"=w910, "Slope"=w904) -> ("Units"=w899:string, "Display Precision"=w903:i32, "Display"=w898:dbl, "VISA session"=w911:refnum<visa-resource-name>, "Available Display Types Out"=w902:string[], "error out"=w909:errorcluster)  [unwired: 4 in, 3 out]
            "Display 3" <- w898
            "Units 3" <- w899
            n110 = property on="Display 3" class="DigNum (strict)"("Precision"=w903) -> ()  [unwired: 2 in, 2 out]
            n111 = call "pref_to_num.vi"("string"=w899) -> ("Numeric"=w901:dbl)
            n112 = property on="Display Type 3" class="Ring (strict)"("Strings []"=w902) -> ()  [unwired: 2 in, 2 out]
            n113 = Multiply(x=w901, y=w898) -> (x*y=w900:dbl)
          }
          frame #8 {
            n114 = local read "Input Mode"() -> (w935:i32)
            n115 = call "SR5110 Read Output"("VISA session (for class)"=w926, "Input Mode"=w935, "Time Constant"=w930, "Display Type"="Display Type copy", "Range"=w929, "error in (no error)"=w928, "Slope"=w931) -> ("Units"=→"Units copy":string, "Display Precision"=w932:i32, "Display"=→"Display copy":dbl, "VISA session"=w925:refnum<visa-resource-name>, "Reference Unlock"=w924:bool, "Available Display Types Out"=w933:string[], "error out"=w927:errorcluster)  [unwired: 4 in, 2 out]
            n116 = property on="Display Type copy" class="Ring (strict)"("Strings []"=w933) -> ()  [unwired: 2 in, 2 out]
            n117 = property on="Display copy" class="DigNum (strict)"("Precision"=w932) -> ()  [unwired: 2 in, 2 out]
          }
          frame #9 {
            n118 = local read "Step  (A)"() -> (w955:dbl)
            n119 = local read "Real start cur"() -> (w956:dbl)
            n120 = Multiply(x=w955, y=w954) -> (x*y=w953:dbl)
            n121 = Add(x=w956, y=w953) -> (x+y=w944:dbl)
            n122 = local read "Real stop cur"() -> (w951:dbl)
            n123 = Greater Or Equal?(x=w944, y=w951) -> (x >= y?=w950:bool)
          }
          frame #10 {
            n124 = call <instrlib>:"KE622x -- Set Current Level.vi"("Resource In"=w965, "Current Level (A) In"=w966, "error in (no error)"=w962) -> ("Resource Out (dupl)"=w963:refnum<visa-resource-name>, "error out"=w964:errorcluster)  [unwired: 11 in]
            n125 = Wait Until Next ms Multiple(millisecond multiple=u32 50) -> ()  [unwired: 1 out]
          }
          frame #11 {
            n126 = Unbundle(w994) -> ("Task out"=w993:i32, "Actual Number of Channels"=w991:u32, "error out"=w992:errorcluster)
            n127 = call <instrlib>:"Data Read Single.vi"("VISA resource name"=w996, "error in (no error)"=w995) -> ("VISA resource name out"=w1002:refnum<visa-resource-name>, "Measurement"=w1004:dbl, "error out"=w1003:errorcluster)  [unwired: 13 in, 2 out]
            n128 = call-poly <userlib>:"DtOLRead.vi"("Number Chan to Read"=w991, "error in (no error)"=w992, "Task in"=w993) -> ("error out"=w989:errorcluster, "2D Data out"=w988:dbl[][], "Task out"=w990:i32)  [unwired: 4 in, 2 out]
            n129 = Index Array(array=w988, index (row) #1=0 ("index (row)"), index (row) #2=1 ("index (row)"), index (row) #3=2 ("index (row)"), index (row) #4=3 ("index (row)"), index (row) #5=4 ("index (row)")) -> (element #1=w987:dbl[], element #2=w981:dbl[], element #3=w980:dbl[], element #4=w979:dbl[], element #5=w978:dbl[])  [unwired: 5 in]
            n130 = Index Array(array=w978, index=0) -> (element=w968:dbl)
            n131 = Index Array(array=w987, index=0) -> (element=w972:dbl)
            n132 = Index Array(array=w981, index=0) -> (element=w971:dbl)
            n133 = Index Array(array=w980, index=0) -> (element=w970:dbl)
            n134 = Index Array(array=w979, index=0) -> (element=w969:dbl)
            n135 = Bundle("Task out"=w990, "error out"=w989) -> (w997:T8)  [unwired: 1 in]
          }
          frame #12 {
          }
        }
        n136 = Build Array (concatenate)(w454, w355) -> (w338:dbl[])
        n137 = property on="TIME GRAPH" class="XYGraph (strict)"("XScale.Mapping Mode"="TIME GRAPH X", "YScale.Mapping Mode"="TIME GRAPH Y") -> ()  [unwired: 2 in, 2 out]
        n138 = property on="MULTIPLE GRAPHS" class="XYGraph (strict)"("XScale.Mapping Mode"="MULTIPLE GRAPHS X", "YScale.Mapping Mode"="MULTIPLE GRAPHS Y") -> ()  [unwired: 2 in, 2 out]
        n139 = Bundle(w340, w246, w247) -> (w199:cluster{dbl, dbl, dbl})  [unwired: 1 in]
        n140 = Unbundle(w199) -> (w243:dbl, w209:dbl, w204:dbl)
        n141 = Unbundle(w199) -> (w184:dbl, w186:dbl, w185:dbl)
        n142 = Multiply(x=w243, y="Current") -> (x*y=w242:dbl)
        n143 = Multiply(x=w204, y="Lock-In, Y") -> (x*y=w205:dbl)
        n144 = Multiply(x=w209, y="Lock-In, X") -> (x*y=w210:dbl)
        n145 = Build Array (concatenate)(w385, w242) -> (w339:dbl[])
        n146 = Build Array (concatenate)(w389, w210) -> (w295:dbl[])
        n147 = Build Array (concatenate)(w388, w205) -> (w294:dbl[])
        n148 = Bundle(w301, w300, w299, w298, w297, "Measurement"=w296) -> (w316:T9)  [unwired: 1 in]
        n149 = Unbundle(w316) -> (w235:dbl, w229:dbl, w224:dbl, w219:dbl, w214:dbl, "Measurement"=w238:dbl)
        n150 = Unbundle(w316) -> (w191:dbl, w190:dbl, w189:dbl, w188:dbl, w187:dbl, "Measurement"=w192:dbl)
        n151 = Format Into String(format string="%08d  %8.2e %12g %14.5e %12.4e %12.4e  %12.4e %12.4e  %12.4e  %12g \\n", initial string=w193, w354, w192, w191, w190, w189, w188, w187, w186, w185, w184) -> ()  [unwired: 1 in, 2 out]
        n152 = Multiply(x=w238, y="2000") -> (x*y=w236:dbl)
        n153 = Multiply(x=w229, y="DAQ A1") -> (x*y=w230:dbl)
        n154 = Multiply(x=w235, y="DAQ A0") -> (x*y=w234:dbl)
        n155 = Multiply(x="DAQ A2", y=w224) -> (x*y=w225:dbl)
        n156 = Multiply(x=w214, y="DAQ A4") -> (x*y=w215:dbl)
        n157 = Multiply(x=w219, y="DAQ A3") -> (x*y=w220:dbl)
        n158 = Build Array (concatenate)(w455, w236) -> (w337:dbl[])
        n159 = Build Array (concatenate)(w343, w234) -> (w336:dbl[])
        n160 = Build Array (concatenate)(w342, w230) -> (w335:dbl[])
        n161 = Build Array (concatenate)(w341, w225) -> (w334:dbl[])
        n162 = Build Array (concatenate)(w445, w220) -> (w333:dbl[])
        n163 = Build Array (concatenate)(w293, w215) -> (w292:dbl[])
        n164 = Bundle(w339, w338, w337, w336, w335, w334, w333, w292, w295, w294) -> (w326:T10)  [unwired: 1 in]
        n165 = Unbundle(w326) -> (w244:dbl[], w202:dbl[], w241:dbl[], w232:dbl[], w227:dbl[], w222:dbl[], w217:dbl[], w211:dbl[], w207:dbl[], w201:dbl[])
        n166 = Bundle(w202, w244) -> (w245:cluster{dbl[], dbl[]})  [unwired: 1 in]
        n167 = Bundle(w202, w241) -> (w240:cluster{dbl[], dbl[]})  [unwired: 1 in]
        n168 = Bundle(w202, w232) -> (w231:cluster{dbl[], dbl[]})  [unwired: 1 in]
        n169 = Bundle(w202, w227) -> (w226:cluster{dbl[], dbl[]})  [unwired: 1 in]
        n170 = Bundle(w202, w217) -> (w216:cluster{dbl[], dbl[]})  [unwired: 1 in]
        n171 = Bundle(w202, w222) -> (w221:cluster{dbl[], dbl[]})  [unwired: 1 in]
        n172 = Bundle(w202, w211) -> (w212:cluster{dbl[], dbl[]})  [unwired: 1 in]
        n173 = Bundle(w202, w207) -> (w206:cluster{dbl[], dbl[]})  [unwired: 1 in]
        n174 = Bundle(w202, w201) -> (w200:cluster{dbl[], dbl[]})  [unwired: 1 in]
        n175 = Build Array(w245, w240, w231, w226, w221, w216, w212, w206, w200) -> (→"TIME GRAPH":cluster{dbl[], dbl[]}[])
        n176 = Unbundle(w326) -> (w325:dbl[], w324:dbl[], w323:dbl[], w322:dbl[], w321:dbl[], w320:dbl[], w319:dbl[], w318:dbl[], w287:dbl[])  [unwired: 1 out]
        n177 = case shown="\"V, Keithley DAQ A3\"" "X-Axis" {
          tunnel: [w475 w517 w552 w580 w622 w657 w692 w717 w752] -> w317
          tunnel: w325 -> [w472 w516 w551 w587 w621 w656 w690 w725 w760]
          tunnel: w324 -> [w489 w507 w550 w586 w620 w655 w689 w724 w759]
          tunnel: w323 -> [w488 w515 w542 w585 w619 w654 w688 w723 w758]
          tunnel: w322 -> [w487 w514 w549 w577 w618 w653 w687 w722 w757]
          tunnel: w321 -> [w486 w513 w548 w584 w612 w652 w686 w721 w756]
          tunnel: w320 -> [w485 w512 w547 w583 w617 w647 w685 w720 w755]
          tunnel: w319 -> [w484 w511 w546 w582 w616 w651 w691 w719 w754]
          tunnel: w318 -> [w483 w510 w545 w581 w615 w650 w684 w726 w753]
          tunnel: w287 -> [w473 w508 w543 w578 w613 w648 w683 w718 w761]
          frame "I, Keithley 6221", Default {
            n178 = Bundle(w472, w489) -> (w482:cluster{dbl[], dbl[]})  [unwired: 1 in]
            n179 = Bundle(w472, w488) -> (w481:cluster{dbl[], dbl[]})  [unwired: 1 in]
            n180 = Bundle(w472, w487) -> (w480:cluster{dbl[], dbl[]})  [unwired: 1 in]
            n181 = Bundle(w472, w486) -> (w479:cluster{dbl[], dbl[]})  [unwired: 1 in]
            n182 = Bundle(w472, w485) -> (w478:cluster{dbl[], dbl[]})  [unwired: 1 in]
            n183 = Bundle(w472, w484) -> (w477:cluster{dbl[], dbl[]})  [unwired: 1 in]
            n184 = Bundle(w472, w483) -> (w476:cluster{dbl[], dbl[]})  [unwired: 1 in]
            n185 = Bundle(w472, w473) -> (w474:cluster{dbl[], dbl[]})  [unwired: 1 in]
            n186 = Build Array(w482, w481, w480, w479, w478, w477, w476, w474) -> (w475:cluster{dbl[], dbl[]}[])
            n187 = property on="MULTIPLE GRAPHS" class="XYGraph (strict)"("XScale.NameLbl.Text"="Keithley 6221, mA" ("X Scale.Name Label.Text")) -> ()  [unwired: 2 in, 2 out]
            n188 = property on="MULTIPLE GRAPHS" class="XYGraph (strict)"("Active Plot"=u32 0, "Plot.Plot Name"="Mult, 2000 V", "Active Plot"=u32 1, "Plot.Plot Name"="DAQ A0", "Active Plot"=u32 2, "Plot.Plot Name"="DAQ A1", "Active Plot"=u32 3, "Plot.Plot Name"="DAQ A2", "Active Plot"=u32 4, "Plot.Plot Name"="DAQ A3", "Active Plot"=u32 5, "Plot.Plot Name"="DAQ A4", "Active Plot"=u32 6, "Plot.Plot Name"="Lock-In, X", "Active Plot"=u32 7, "Plot.Plot Name"="Lock-In, Y") -> ()  [unwired: 2 in, 2 out]
          }
          frame "V, Keithley 2000" {
            n189 = property on="MULTIPLE GRAPHS" class="XYGraph (strict)"("XScale.NameLbl.Text"="Keithley 2000, V" ("X Scale.Name Label.Text")) -> ()  [unwired: 2 in, 2 out]
            n190 = Bundle(w507, w516) -> (w524:cluster{dbl[], dbl[]})  [unwired: 1 in]
            n191 = Bundle(w507, w515) -> (w523:cluster{dbl[], dbl[]})  [unwired: 1 in]
            n192 = Bundle(w507, w514) -> (w522:cluster{dbl[], dbl[]})  [unwired: 1 in]
            n193 = Bundle(w507, w513) -> (w521:cluster{dbl[], dbl[]})  [unwired: 1 in]
            n194 = Bundle(w507, w512) -> (w520:cluster{dbl[], dbl[]})  [unwired: 1 in]
            n195 = Bundle(w507, w511) -> (w519:cluster{dbl[], dbl[]})  [unwired: 1 in]
            n196 = Bundle(w507, w510) -> (w518:cluster{dbl[], dbl[]})  [unwired: 1 in]
            n197 = Bundle(w507, w508) -> (w509:cluster{dbl[], dbl[]})  [unwired: 1 in]
            n198 = Build Array(w524, w523, w522, w521, w520, w519, w518, w509) -> (w517:cluster{dbl[], dbl[]}[])
            n199 = property on="MULTIPLE GRAPHS" class="XYGraph (strict)"("Active Plot"=u32 0, "Plot.Plot Name"="I, 6221 mA", "Active Plot"=u32 1, "Plot.Plot Name"="DAQ A0", "Active Plot"=u32 2, "Plot.Plot Name"="DAQ A1", "Active Plot"=u32 3, "Plot.Plot Name"="DAQ A2", "Active Plot"=u32 4, "Plot.Plot Name"="DAQ A3", "Active Plot"=u32 5, "Plot.Plot Name"="DAQ A4", "Active Plot"=u32 6, "Plot.Plot Name"="Lock-In, X", "Active Plot"=u32 7, "Plot.Plot Name"="Lock-In, Y") -> ()  [unwired: 2 in, 2 out]
          }
          frame "V, Keithley DAQ A0" {
            n200 = property on="MULTIPLE GRAPHS" class="XYGraph (strict)"("XScale.NameLbl.Text"="Keithley DAQ A0, V" ("X Scale.Name Label.Text")) -> ()  [unwired: 2 in, 2 out]
            n201 = Bundle(w542, w543) -> (w544:cluster{dbl[], dbl[]})  [unwired: 1 in]
            n202 = Bundle(w542, w551) -> (w559:cluster{dbl[], dbl[]})  [unwired: 1 in]
            n203 = Bundle(w542, w550) -> (w558:cluster{dbl[], dbl[]})  [unwired: 1 in]
            n204 = Bundle(w542, w549) -> (w557:cluster{dbl[], dbl[]})  [unwired: 1 in]
            n205 = Bundle(w542, w548) -> (w556:cluster{dbl[], dbl[]})  [unwired: 1 in]
            n206 = Bundle(w542, w547) -> (w555:cluster{dbl[], dbl[]})  [unwired: 1 in]
            n207 = Bundle(w542, w546) -> (w554:cluster{dbl[], dbl[]})  [unwired: 1 in]
            n208 = Bundle(w542, w545) -> (w553:cluster{dbl[], dbl[]})  [unwired: 1 in]
            n209 = Build Array(w559, w558, w557, w556, w555, w554, w553, w544) -> (w552:cluster{dbl[], dbl[]}[])
            n210 = property on="MULTIPLE GRAPHS" class="XYGraph (strict)"("Active Plot"=u32 0, "Plot.Plot Name"="I, 6221 mA", "Active Plot"=u32 1, "Plot.Plot Name"="Mult, 2000 V", "Active Plot"=u32 2, "Plot.Plot Name"="DAQ A1", "Active Plot"=u32 3, "Plot.Plot Name"="DAQ A2", "Active Plot"=u32 4, "Plot.Plot Name"="DAQ A3", "Active Plot"=u32 5, "Plot.Plot Name"="DAQ A4", "Active Plot"=u32 6, "Plot.Plot Name"="Lock-In, X", "Active Plot"=u32 7, "Plot.Plot Name"="Lock-In, Y") -> ()  [unwired: 2 in, 2 out]
          }
          frame "V, Keithley DAQ A1" {
            n211 = property on="MULTIPLE GRAPHS" class="XYGraph (strict)"("XScale.NameLbl.Text"="Keithley DAQ A1, V" ("X Scale.Name Label.Text")) -> ()  [unwired: 2 in, 2 out]
            n212 = Bundle(w577, w587) -> (w589:cluster{dbl[], dbl[]})  [unwired: 1 in]
            n213 = Bundle(w577, w586) -> (w590:cluster{dbl[], dbl[]})  [unwired: 1 in]
            n214 = Bundle(w577, w585) -> (w591:cluster{dbl[], dbl[]})  [unwired: 1 in]
            n215 = Bundle(w577, w584) -> (w592:cluster{dbl[], dbl[]})  [unwired: 1 in]
            n216 = Bundle(w577, w583) -> (w593:cluster{dbl[], dbl[]})  [unwired: 1 in]
            n217 = Bundle(w577, w582) -> (w594:cluster{dbl[], dbl[]})  [unwired: 1 in]
            n218 = Bundle(w577, w581) -> (w595:cluster{dbl[], dbl[]})  [unwired: 1 in]
            n219 = Bundle(w577, w578) -> (w579:cluster{dbl[], dbl[]})  [unwired: 1 in]
            n220 = Build Array(w589, w590, w591, w592, w593, w594, w595, w579) -> (w580:cluster{dbl[], dbl[]}[])
            n221 = property on="MULTIPLE GRAPHS" class="XYGraph (strict)"("Active Plot"=u32 0, "Plot.Plot Name"="I, 6221 mA", "Active Plot"=u32 1, "Plot.Plot Name"="Mult, 2000 V", "Active Plot"=u32 2, "Plot.Plot Name"="DAQ A0", "Active Plot"=u32 3, "Plot.Plot Name"="DAQ A2", "Active Plot"=u32 4, "Plot.Plot Name"="DAQ A3", "Active Plot"=u32 5, "Plot.Plot Name"="DAQ A4", "Active Plot"=u32 6, "Plot.Plot Name"="Lock-In, X", "Active Plot"=u32 7, "Plot.Plot Name"="Lock-In, Y") -> ()  [unwired: 2 in, 2 out]
          }
          frame "V, Keithley DAQ A2" {
            n222 = property on="MULTIPLE GRAPHS" class="XYGraph (strict)"("XScale.NameLbl.Text"="Keithley DAQ A2, V" ("X Scale.Name Label.Text")) -> ()  [unwired: 2 in, 2 out]
            n223 = Bundle(w612, w621) -> (w623:cluster{dbl[], dbl[]})  [unwired: 1 in]
            n224 = Bundle(w612, w620) -> (w624:cluster{dbl[], dbl[]})  [unwired: 1 in]
            n225 = Bundle(w612, w619) -> (w625:cluster{dbl[], dbl[]})  [unwired: 1 in]
            n226 = Bundle(w612, w618) -> (w626:cluster{dbl[], dbl[]})  [unwired: 1 in]
            n227 = Bundle(w612, w617) -> (w627:cluster{dbl[], dbl[]})  [unwired: 1 in]
            n228 = Bundle(w612, w616) -> (w628:cluster{dbl[], dbl[]})  [unwired: 1 in]
            n229 = Bundle(w612, w615) -> (w629:cluster{dbl[], dbl[]})  [unwired: 1 in]
            n230 = Bundle(w612, w613) -> (w614:cluster{dbl[], dbl[]})  [unwired: 1 in]
            n231 = Build Array(w623, w624, w625, w626, w627, w628, w629, w614) -> (w622:cluster{dbl[], dbl[]}[])
            n232 = property on="MULTIPLE GRAPHS" class="XYGraph (strict)"("Active Plot"=u32 0, "Plot.Plot Name"="I, 6221 mA", "Active Plot"=u32 1, "Plot.Plot Name"="Mult, 2000 V", "Active Plot"=u32 2, "Plot.Plot Name"="DAQ A0", "Active Plot"=u32 3, "Plot.Plot Name"="DAQ A1", "Active Plot"=u32 4, "Plot.Plot Name"="DAQ A3", "Active Plot"=u32 5, "Plot.Plot Name"="DAQ A4", "Active Plot"=u32 6, "Plot.Plot Name"="Lock-In, X", "Active Plot"=u32 7, "Plot.Plot Name"="Lock-In, Y") -> ()  [unwired: 2 in, 2 out]
          }
          frame "V, Keithley DAQ A3" {
            n233 = property on="MULTIPLE GRAPHS" class="XYGraph (strict)"("XScale.NameLbl.Text"="Keithley DAQ A3, V" ("X Scale.Name Label.Text")) -> ()  [unwired: 2 in, 2 out]
            n234 = Bundle(w647, w656) -> (w658:cluster{dbl[], dbl[]})  [unwired: 1 in]
            n235 = Bundle(w647, w655) -> (w659:cluster{dbl[], dbl[]})  [unwired: 1 in]
            n236 = Bundle(w647, w654) -> (w660:cluster{dbl[], dbl[]})  [unwired: 1 in]
            n237 = Bundle(w647, w653) -> (w661:cluster{dbl[], dbl[]})  [unwired: 1 in]
            n238 = Bundle(w647, w652) -> (w662:cluster{dbl[], dbl[]})  [unwired: 1 in]
            n239 = Bundle(w647, w651) -> (w663:cluster{dbl[], dbl[]})  [unwired: 1 in]
            n240 = Bundle(w647, w650) -> (w664:cluster{dbl[], dbl[]})  [unwired: 1 in]
            n241 = Bundle(w647, w648) -> (w649:cluster{dbl[], dbl[]})  [unwired: 1 in]
            n242 = Build Array(w658, w659, w660, w661, w662, w663, w664, w649) -> (w657:cluster{dbl[], dbl[]}[])
            n243 = property on="MULTIPLE GRAPHS" class="XYGraph (strict)"("Active Plot"=u32 0, "Plot.Plot Name"="I, 6221 mA", "Active Plot"=u32 1, "Plot.Plot Name"="Mult, 2000 V", "Active Plot"=u32 2, "Plot.Plot Name"="DAQ A0", "Active Plot"=u32 3, "Plot.Plot Name"="DAQ A1", "Active Plot"=u32 4, "Plot.Plot Name"="DAQ A2", "Active Plot"=u32 5, "Plot.Plot Name"="DAQ A4", "Active Plot"=u32 6, "Plot.Plot Name"="Lock-In, X", "Active Plot"=u32 7, "Plot.Plot Name"="Lock-In,Y") -> ()  [unwired: 2 in, 2 out]
          }
          frame "V, Keithley DAQ A4" {
            n244 = property on="MULTIPLE GRAPHS" class="XYGraph (strict)"("XScale.NameLbl.Text"="Keithley DAQ A4, V" ("X Scale.Name Label.Text")) -> ()  [unwired: 2 in, 2 out]
            n245 = Bundle(w691, w690) -> (w694:cluster{dbl[], dbl[]})  [unwired: 1 in]
            n246 = Bundle(w691, w689) -> (w695:cluster{dbl[], dbl[]})  [unwired: 1 in]
            n247 = Bundle(w691, w688) -> (w696:cluster{dbl[], dbl[]})  [unwired: 1 in]
            n248 = Bundle(w691, w687) -> (w697:cluster{dbl[], dbl[]})  [unwired: 1 in]
            n249 = Bundle(w691, w686) -> (w698:cluster{dbl[], dbl[]})  [unwired: 1 in]
            n250 = Bundle(w691, w685) -> (w699:cluster{dbl[], dbl[]})  [unwired: 1 in]
            n251 = Bundle(w691, w684) -> (w700:cluster{dbl[], dbl[]})  [unwired: 1 in]
            n252 = Bundle(w691, w683) -> (w693:cluster{dbl[], dbl[]})  [unwired: 1 in]
            n253 = Build Array(w694, w695, w696, w697, w698, w699, w700, w693) -> (w692:cluster{dbl[], dbl[]}[])
            n254 = property on="MULTIPLE GRAPHS" class="XYGraph (strict)"("Active Plot"=u32 0, "Plot.Plot Name"="I, 6221 mA", "Active Plot"=u32 1, "Plot.Plot Name"="Mult, 2000 V", "Active Plot"=u32 2, "Plot.Plot Name"="DAQ A0", "Active Plot"=u32 3, "Plot.Plot Name"="DAQ A1", "Active Plot"=u32 4, "Plot.Plot Name"="DAQ A2", "Active Plot"=u32 5, "Plot.Plot Name"="DAQ A3", "Active Plot"=u32 6, "Plot.Plot Name"="Lock-In, X", "Active Plot"=u32 7, "Plot.Plot Name"="Lock-In, Y") -> ()  [unwired: 2 in, 2 out]
          }
          frame "V, Lock-In X" {
            n255 = property on="MULTIPLE GRAPHS" class="XYGraph (strict)"("XScale.NameLbl.Text"="Lock-In X, V" ("X Scale.Name Label.Text")) -> ()  [unwired: 2 in, 2 out]
            n256 = Bundle(w726, w725) -> (w728:cluster{dbl[], dbl[]})  [unwired: 1 in]
            n257 = Bundle(w726, w724) -> (w729:cluster{dbl[], dbl[]})  [unwired: 1 in]
            n258 = Bundle(w726, w723) -> (w730:cluster{dbl[], dbl[]})  [unwired: 1 in]
            n259 = Bundle(w726, w722) -> (w731:cluster{dbl[], dbl[]})  [unwired: 1 in]
            n260 = Bundle(w726, w721) -> (w732:cluster{dbl[], dbl[]})  [unwired: 1 in]
            n261 = Bundle(w726, w720) -> (w733:cluster{dbl[], dbl[]})  [unwired: 1 in]
            n262 = Bundle(w726, w719) -> (w734:cluster{dbl[], dbl[]})  [unwired: 1 in]
            n263 = Bundle(w726, w718) -> (w727:cluster{dbl[], dbl[]})  [unwired: 1 in]
            n264 = Build Array(w728, w729, w730, w731, w732, w733, w734, w727) -> (w717:cluster{dbl[], dbl[]}[])
            n265 = property on="MULTIPLE GRAPHS" class="XYGraph (strict)"("Active Plot"=u32 0, "Plot.Plot Name"="I, 6221 mA", "Active Plot"=u32 1, "Plot.Plot Name"="Mult, 2000 V", "Active Plot"=u32 2, "Plot.Plot Name"="DAQ A0", "Active Plot"=u32 3, "Plot.Plot Name"="DAQ A1", "Active Plot"=u32 4, "Plot.Plot Name"="DAQ A2", "Active Plot"=u32 5, "Plot.Plot Name"="DAQ A3", "Active Plot"=u32 6, "Plot.Plot Name"="DAQ A4", "Active Plot"=u32 7, "Plot.Plot Name"="Lock-In, Y") -> ()  [unwired: 2 in, 2 out]
          }
          frame "V, Lock-In Y" {
            n266 = property on="MULTIPLE GRAPHS" class="XYGraph (strict)"("XScale.NameLbl.Text"="Lock-In Y, V" ("X Scale.Name Label.Text")) -> ()  [unwired: 2 in, 2 out]
            n267 = Bundle(w761, w760) -> (w769:cluster{dbl[], dbl[]})  [unwired: 1 in]
            n268 = Bundle(w761, w759) -> (w768:cluster{dbl[], dbl[]})  [unwired: 1 in]
            n269 = Bundle(w761, w758) -> (w767:cluster{dbl[], dbl[]})  [unwired: 1 in]
            n270 = Bundle(w761, w757) -> (w766:cluster{dbl[], dbl[]})  [unwired: 1 in]
            n271 = Bundle(w761, w756) -> (w765:cluster{dbl[], dbl[]})  [unwired: 1 in]
            n272 = Bundle(w761, w755) -> (w764:cluster{dbl[], dbl[]})  [unwired: 1 in]
            n273 = Bundle(w761, w754) -> (w763:cluster{dbl[], dbl[]})  [unwired: 1 in]
            n274 = Bundle(w761, w753) -> (w762:cluster{dbl[], dbl[]})  [unwired: 1 in]
            n275 = Build Array(w769, w768, w767, w766, w765, w764, w763, w762) -> (w752:cluster{dbl[], dbl[]}[])
            n276 = property on="MULTIPLE GRAPHS" class="XYGraph (strict)"("Active Plot"=u32 0, "Plot.Plot Name"="I, 6221 mA", "Active Plot"=u32 1, "Plot.Plot Name"="Mult, 2000 V", "Active Plot"=u32 2, "Plot.Plot Name"="DAQ A0", "Active Plot"=u32 3, "Plot.Plot Name"="DAQ A1", "Active Plot"=u32 4, "Plot.Plot Name"="DAQ A2", "Active Plot"=u32 5, "Plot.Plot Name"="DAQ A3", "Active Plot"=u32 6, "Plot.Plot Name"="DAQ A4", "Active Plot"=u32 7, "Plot.Plot Name"="Lock-In, X") -> ()  [unwired: 2 in, 2 out]
          }
        }
        "MULTIPLE GRAPHS" <- w317
        n277 = Unbundle(w326) -> (w332:dbl[], w331:dbl[], w330:dbl[], w329:dbl[], w328:dbl[], w327:dbl[], w288:dbl[], w289:dbl[], w290:dbl[], w291:dbl[])
        n278 = Multiply(x="Time Delay", y=u16 1000) -> (x*y=w183:u16)
        n279 = Wait Until Next ms Multiple(millisecond multiple=w183) -> ()  [unwired: 1 out]
        "2000" <- w438
        "DAQ A0" <- w301
        "DAQ A1" <- w300
        "DAQ A2" <- w299
        "DAQ A3" <- w298
        "DAQ A4" <- w297
      }
    }
    frame #3 {
      # "Closing instrumental \nconnections"
      n280 = Unbundle(w1021) -> ("Task out"=w1020:i32, "error out"=w1019:errorcluster)
      n281 = call <instrlib>:"Close.vi"("VISA resource name"=w1026, "error in (no error)"=w1027) -> ()  [unwired: 17 in, 1 out]
      n282 = call "SR51XX Close"("error in (no error)"=w1022, "VISA session"=w1023) -> ()  [unwired: 1 out]
      n283 = call <instrlib>:"Close.vi"("VISA resource name"=w1024, "error in (no error)"=w1025) -> ()  [unwired: 13 in, 1 out]
      n284 = call <userlib>:"DtOLCloseTask.vi"("Error in"=w1019, "Task in"=w1020) -> ("Error Out"=w1028:errorcluster)  [unwired: 9 in]
      n285 = call <vilib>:"Simple Error Handler.vi"("error in (no error)"=w1028) -> ()  [unwired: 4 in, 5 out]
    }
  }
